vi "AcquireImage.vi"(5 "External display":bool, 6 "Image Conversion":string, 7 "measure call context in":refnum<class "Measure Call Context.lvclass">, 8 "error in (no error)":errorcluster, 9 "Buffer Number Out in":u32, 10 "Accessor:Is Canceled":bool, 11 "Refnum in":T2) -> (0 "error out":errorcluster, 1 "Valid Result":bool, 2 "Measurement Results":T1, 3 "Buffer Number Out out":u32)   [LabVIEW 2021, in "ImageStreamRendering.lvlib"]
uses:
  ImageStreamRendering.lvlib
  <vilib>/userdefined/High Color/IMAQdx.ctl
  <vilib>/MeasurementLink/MeasurementLink Measurement Server/Measure Call Context/Measure Call Context.lvclass
  Measurement Results.ctl
  <resource>/objmgr/imaqdx.rc
  <vilib>/vision/driver/NI_Vision_Acquisition_Software.lvlib
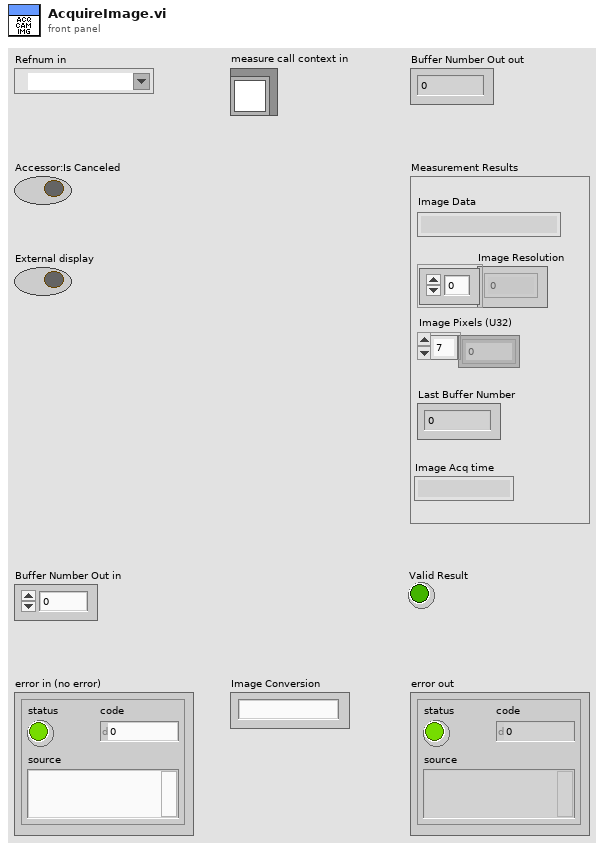
[diagram p1: front panel]
types:
  T1 = typedef "ImageStreamRendering.lvlib/Measurement Results.ctl" = cluster{"Image Data":string, "Image Resolution":i32[], "Image Pixels (U32)":u32[], "Last Buffer Number":u32, "Image Acq time":string}
  T2 = typedef "IMAQdx.ctl" = refnum<k21>
  T3 = typedef "IMAQ Image.ctl" = refnum<image>
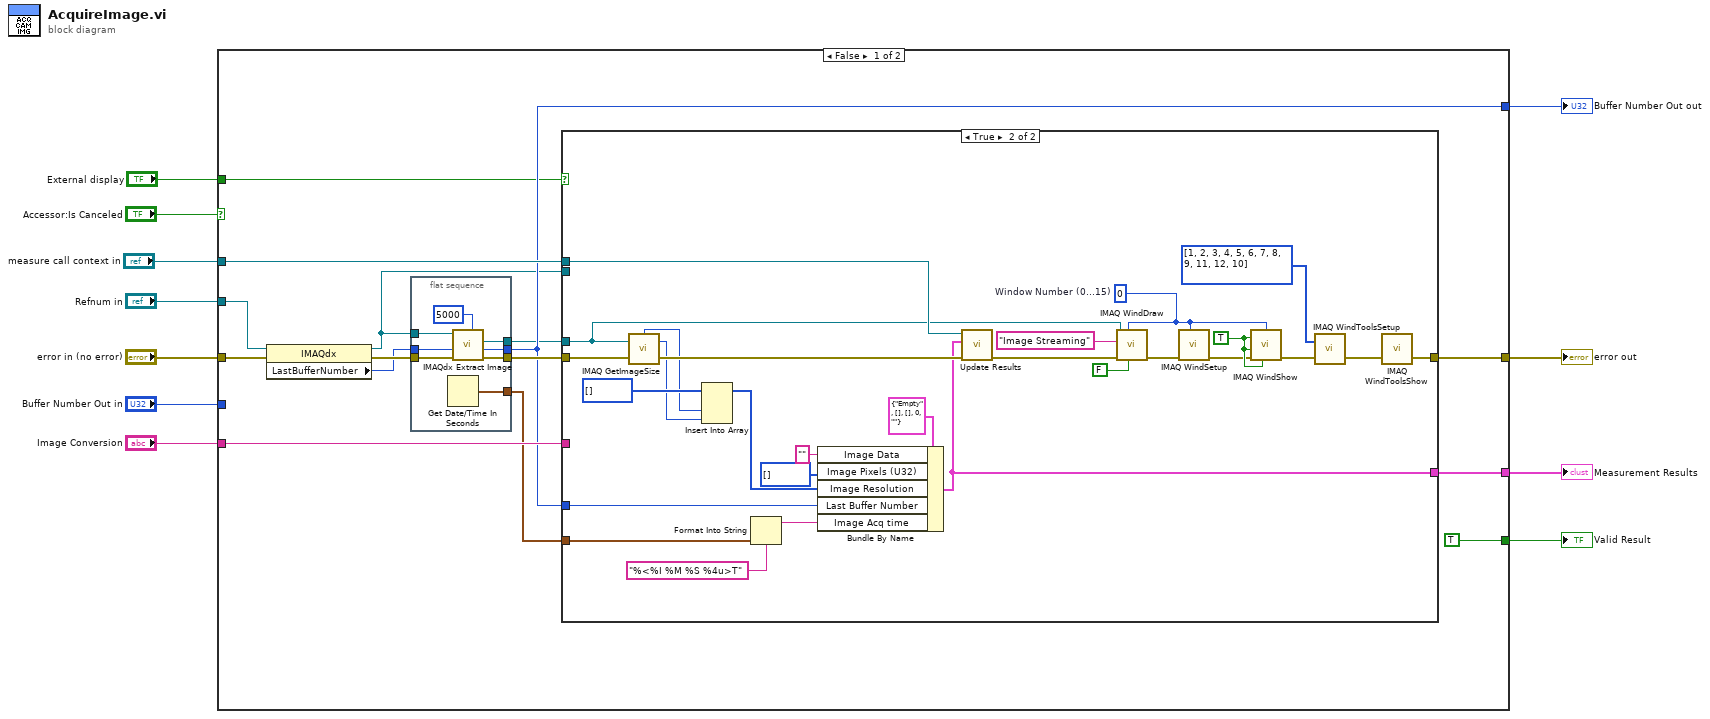
[diagram p0: block diagram]
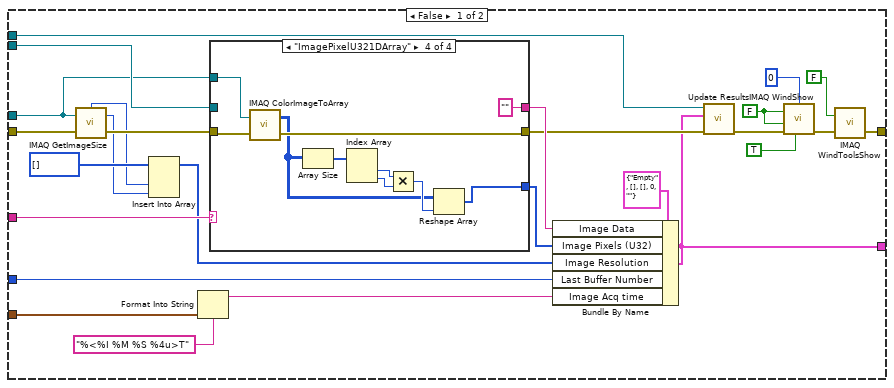
[diagram p2: hidden frame]
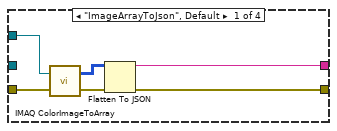
[diagram p3: hidden frame]
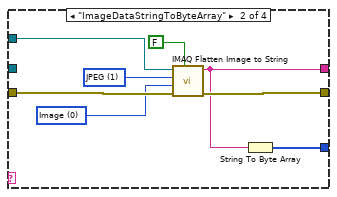
[diagram p4: hidden frame]
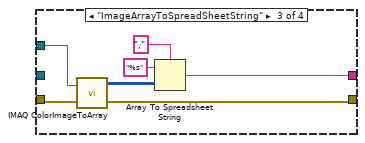
[diagram p5: hidden frame]
diagram:
  n1 = case shown="False" "Accessor:Is Canceled" {
    tunnel: "Refnum in" -> [w26 _]
    tunnel: [w13 w119] -> w7
    tunnel: [w18 w120] -> w8
    tunnel: "Buffer Number Out in" -> [_ w120]
    tunnel: "error in (no error)" -> [w23 w119]
    tunnel: "Image Conversion" -> [w22 _]
    tunnel: [w16 _] -> w3
    tunnel: "measure call context in" -> [w21 _]
    tunnel: [TRUE _] -> w2
    tunnel: "External display" -> [w12 _]
    frame False {
      n2 = property class="IMAQdx"(reference=w26, error in=w23) -> (reference out=w15:T2, error out=w25:errorcluster, "LastBufferNumber"=w24:u32)
      n3 = flat-sequence {
        tunnel: w15 -> [w118]
        tunnel: w25 -> [w117]
        tunnel: w24 -> [w116]
        tunnel: [w114] -> w19
        tunnel: [w113] -> w14
        tunnel: [w112] -> w18
        tunnel: [w111] -> w17
        frame #0 {
          n4 = Get Date/Time In Seconds() -> (seconds since 1Jan1904=w111:timestamp)
          n5 = call <vilib>:"IMAQdx Extract Image.vi"("Timeout (ms)"=5000, "error in"=w117, "Buffer Number In"=w116, "Session In"=w118) -> ("error out"=w114:errorcluster, "Buffer Number Out"=w112:u32, "Image Out"=w113:T3)  [unwired: 4 in, 1 out]
        }
      }
      n6 = case shown="True" w12 {
        tunnel: w22 -> [w52 _]
        tunnel: w21 -> [w51 w97]
        tunnel: w19 -> [w47 w109]
        tunnel: w18 -> [w40 w103]
        tunnel: w17 -> [w39 w102]
        tunnel: [w36 w96] -> w16
        tunnel: w15 -> [w35 _]
        tunnel: w14 -> [w34 w94]
        tunnel: [w27 w88] -> w13
        frame False {
          w31 = FALSE ("Hide/Show (Show)")
          n7 = call "IMAQ GetImageSize"("Image"=w34, "error in (no error)"=w47) -> ("Y Resolution"=w42:i32, "X Resolution"=w43:i32, "error out"=w46:errorcluster)  [unwired: 2 in]
          n8 = Insert Into Array(array=i32[] [] ("size(s)"), new element #1=w43, new element #2=w42) -> (w41:i32[])  [unwired: 1 in]
          n9 = Format Into String(format string="%<%I %M %S %4u>T", w39) -> (resulting string=w37:string)  [unwired: 2 in, 1 out]
          n10 = case shown="\"ImagePixelU321DArray\"" w52 {
            tunnel: w46 -> [w58 w66 w73 w83]
            tunnel: [w56 w65 w72 w82] -> w45
            tunnel: [w55 w59 w69 "" ("spreadsheet string")] -> w49
            tunnel: w34 -> [w53 w60 w67 w80]
            tunnel: [_ w63 _ w74] -> w48
            tunnel: w35 -> [_ _ _ _]
            frame "ImageArrayToJson", Default {
              n11 = call "IMAQ ColorImageToArray"("Image"=w53, "error in (no error)"=w58) -> ("Image Pixels (U32)"=w54:u32[][], "error out"=w57:errorcluster)  [unwired: 2 in, 1 out]
              n12 = Flatten To JSON(anything=w54, error in (no error)=w57) -> (JSON string=w55:string, 11:w56:errorcluster)  [unwired: 1 in]
            }
            frame "ImageDataStringToByteArray" {
              w62 = 1 items=["None", "JPEG", "PACKED BINARY"] ("Compression (None)")
              w64 = 0 items=["Image", "Image and Vision Info", "Reference to Image"] ("Type of Flatten (Image and Vision Info)")
              n13 = call "IMAQ Flatten Image to String"("Flatten with Process-Unique Name (F)"=FALSE, "error in (no error)"=w66, "Type of Flatten (Image and Vision Info)"=w64, "Compression (None)"=w62, "Image"=w60) -> ("error out"=w65:errorcluster, "Data String"=w59:string)  [unwired: 5 in]
              n14 = String To Byte Array(string=w59) -> (unsigned byte array=w63:u8[])
            }
            frame "ImageArrayToSpreadSheetString" {
              n15 = call "IMAQ ColorImageToArray"("Image"=w67, "error in (no error)"=w73) -> ("Image Pixels (U32)"=w71:u32[][], "error out"=w72:errorcluster)  [unwired: 2 in, 1 out]
              n16 = Array To Spreadsheet String(delimiter (Tab)=",", array=w71, 3:"%s" ("format string")) -> (spreadsheet string=w69:string)
            }
            frame "ImagePixelU321DArray" {
              n17 = call "IMAQ ColorImageToArray"("Image"=w80, "error in (no error)"=w83) -> ("Image Pixels (U32)"=w76:u32[][], "error out"=w82:errorcluster)  [unwired: 2 in, 1 out]
              n18 = Array Size(array=w76) -> (size(s)=w75:i32[])
              n19 = Index Array(array=w75) -> (element #1=w79:i32, element #2=w78:i32)  [unwired: 2 in]
              n20 = Multiply(x=w79, y=w78) -> (x*y=w77:i32)
              n21 = Reshape Array(w76, w77) -> (w74:u32[])
            }
          }
          n22 = Bundle By Name(cluster=T1 {"Image Data"="Empty", "Image Resolution"=[], "Image Pixels (U32)"=[], "Last Buffer Number"=0, "Image Acq time"=""} ("Measurement Results"), "Image Data"=w49, "Image Pixels (U32)"=w48, "Image Resolution"=w41, "Last Buffer Number"=w40, "Image Acq time"=w37) -> (w36:T1)
          n23 = call <vilib>:"Update Results.vi"("error in"=w45, "measurement results"=w36, "measure call context in"=w51) -> ("error out"=w33:errorcluster)  [unwired: 7 in, 1 out]
          n24 = call "IMAQ WindShow"("error in (no error)"=w33, "Bring To Front? (N)"=w31, "Get/Set Status? (Set)"=TRUE, "Hide/Show (Show)"=w31, "Window Number (0...15)"=0) -> ("error out"=w29:errorcluster)  [unwired: 1 in, 2 out]
          n25 = call "IMAQ WindToolsShow"("Hide/Show (Show)"=FALSE, "error in (no error)"=w29) -> ("error out"=w27:errorcluster)  [unwired: 3 in, 1 out]
        }
        frame True {
          w92 = u32[] [1, 2, 3, 4, 5, 6, 7, 8, 9, 11, 12, 10] items=["No Selection", "Point", "Line", "Rectangle", "Oval", "Polygon", "Freehand Region", "Annulus", "Zoom", "Pan", "Broken Line", "Freehand Line", "Rotated Rectangle"] ("Tools")
          w85 = 0  # Window Number (0...15)
          w93 = TRUE ("Bring To Front? (N)")
          n26 = call "IMAQ GetImageSize"("Image"=w94, "error in (no error)"=w109) -> ("Y Resolution"=w105:i32, "X Resolution"=w106:i32, "error out"=w108:errorcluster)  [unwired: 2 in]
          n27 = Insert Into Array(array=i32[] [] ("size(s)"), new element #1=w106, new element #2=w105) -> (w104:i32[])  [unwired: 1 in]
          n28 = Format Into String(format string="%<%I %M %S %4u>T", w102) -> (resulting string=w100:string)  [unwired: 2 in, 1 out]
          n29 = Bundle By Name(cluster=T1 {"Image Data"="Empty", "Image Resolution"=[], "Image Pixels (U32)"=[], "Last Buffer Number"=0, "Image Acq time"=""} ("Measurement Results"), "Image Data"="", "Image Pixels (U32)"=u32[] [], "Image Resolution"=w104, "Last Buffer Number"=w103, "Image Acq time"=w100) -> (w96:T1)
          n30 = call <vilib>:"Update Results.vi"("error in"=w108, "measurement results"=w96, "measure call context in"=w97) -> ("error out"=w91:errorcluster)  [unwired: 7 in, 1 out]
          n31 = call "IMAQ WindDraw"("Resize to Image Size? (Y)"=FALSE, "Window Number (0...15)"=w85, "error in (no error)"=w91, "Title"="Image Streaming", "Image"=w94) -> ("error out"=w87:errorcluster)  [unwired: 5 in, 1 out]
          n32 = call "IMAQ WindSetup"("Window Number (0...15)"=w85, "error in (no error)"=w87) -> ("error out"=w86:errorcluster)  [unwired: 9 in]
          n33 = call "IMAQ WindShow"("error in (no error)"=w86, "Bring To Front? (N)"=w93, "Get/Set Status? (Set)"=w93, "Hide/Show (Show)"=w93, "Window Number (0...15)"=w85) -> ("error out"=w90:errorcluster)  [unwired: 1 in, 2 out]
          n34 = call "IMAQ WindToolsSetup"("Tools"=w92, "error in (no error)"=w90) -> ("error out"=w89:errorcluster)  [unwired: 4 in]
          n35 = call "IMAQ WindToolsShow"("error in (no error)"=w89) -> ("error out"=w88:errorcluster)  [unwired: 4 in, 1 out]
        }
      }
    }
    frame True {
    }
  }
  "Buffer Number Out out" <- w8
  "error out" <- w7
  "Measurement Results" <- w3
  "Valid Result" <- w2
